vi "UpdateHistory.vi"(4 "Description":string, 5 "LibraryPK":i32, 6 "Library":string, 7 "Action":string, 8 "error in (no error)":errorcluster, 9 "ErrorText":string, 10 "ErrorCode":i32, 11 "Connection in":refnum<class "Connection.lvclass">) -> (0 "error out":errorcluster, 3 "Connection out":refnum<class "Connection.lvclass">)   [LabVIEW 2021, in "ErrorDefinitionSQLite.lvclass"]
uses:
  ErrorDefinitionSQLite.lvclass
  <vilib>/drjdpowell/SQLite Library/SQL Connection/Connection.lvclass
  <vilib>/drjdpowell/SQLite Library/SQL Connection/Execute SQL.vi
  <vilib>/drjdpowell/SQLite Library/SQLite.lvlib
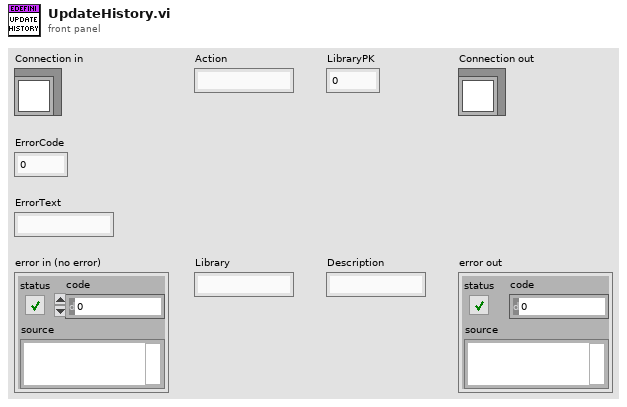
[diagram p1: front panel]
types:
  T1 = cluster{"Action":string, "App.UserName":string, string, "ErrorText":string, "Library":string, "Description":string, string}
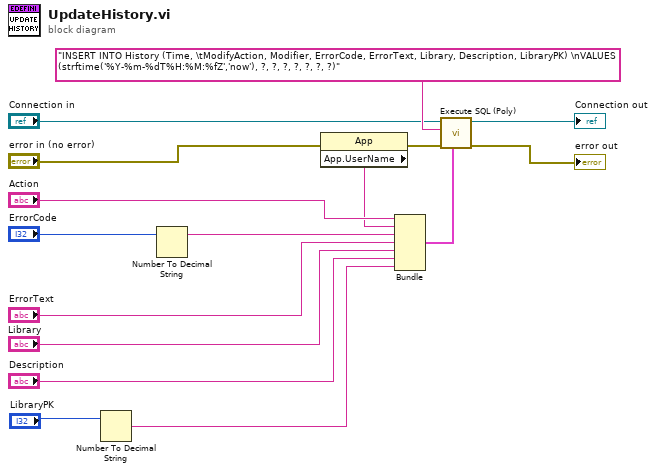
[diagram p0: block diagram]
diagram:
  n1 = Number To Decimal String(number="LibraryPK") -> (decimal integer string=w1:string)  [unwired: 1 in]
  n2 = Number To Decimal String(number="ErrorCode") -> (decimal integer string=w4:string)  [unwired: 1 in]
  n3 = property class="App"(error in="error in (no error)") -> (error out=w12:errorcluster, "App.UserName"=w9:string)  [unwired: 1 in, 1 out]
  n4 = Bundle("Action"="Action", "App.UserName"=w9, w4, "ErrorText"="ErrorText", "Library"="Library", "Description"="Description", w1) -> (w10:T1)  [unwired: 1 in]
  n5 = call-poly <vilib>:"Execute SQL (Poly).vi"("Parameter(s)"=w10, "error in (no error)"=w12, "SQL"="INSERT INTO History (Time, \tModifyAction, Modifier, ErrorCode, ErrorText, Library, Description, LibraryPK) \nVALUES (strftime('%Y-%m-%dT%H:%M:%fZ','now'), ?, ?, ?, ?, ?, ?, ?)", "SQLite Connection in"="Connection in") -> ("error out"=→"error out":errorcluster, "SQLite Connection"=→"Connection out":refnum<class "Connection.lvclass">)  [unwired: 4 in, 2 out]
